vi "Get Username.vi"(0 "Name":T1) -> (4 "Full name":string)   [LabVIEW 2021, in "Reusables.lvlib"]
uses:
  controls/Username.ctl
  Reusables.lvlib
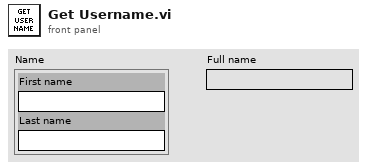
[diagram p1: front panel]
types:
  T1 = typedef "Reusables.lvlib/Username.ctl" = cluster{"First name":string, "Last name":string}
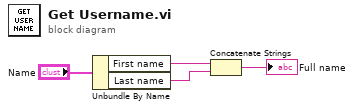
[diagram p0: block diagram]
diagram:
  n1 = Unbundle By Name("Name") -> ("First name"=w3:string, "Last name"=w2:string)
  n2 = Concatenate Strings(w3, w2) -> (→"Full name":string)
